vi "例7-1.vi"() -> ()   [LabVIEW 2017]
panel:
  out "7（X0=10，dx=2，Y）多条曲线":cluster{i32, i32, cluster{dbl[]}[]}(graph)
  out "6（X0=10，dx=2，Y）多条曲线":cluster{i32, i32, dbl[][]}(graph)
  out "5（X0=10，dx=2，Y）多条曲线":cluster{i32, i32, dbl[]}[](graph)
  out "4（X0=10，dx=2，Y）单条曲线":cluster{i32, i32, dbl[]}(graph)
  out "3(Y)多条曲线":cluster{dbl[]}[](graph)
  out "2(Y)多条曲线":dbl[][](graph)
  out "1(Y)单条曲线":dbl[](graph)
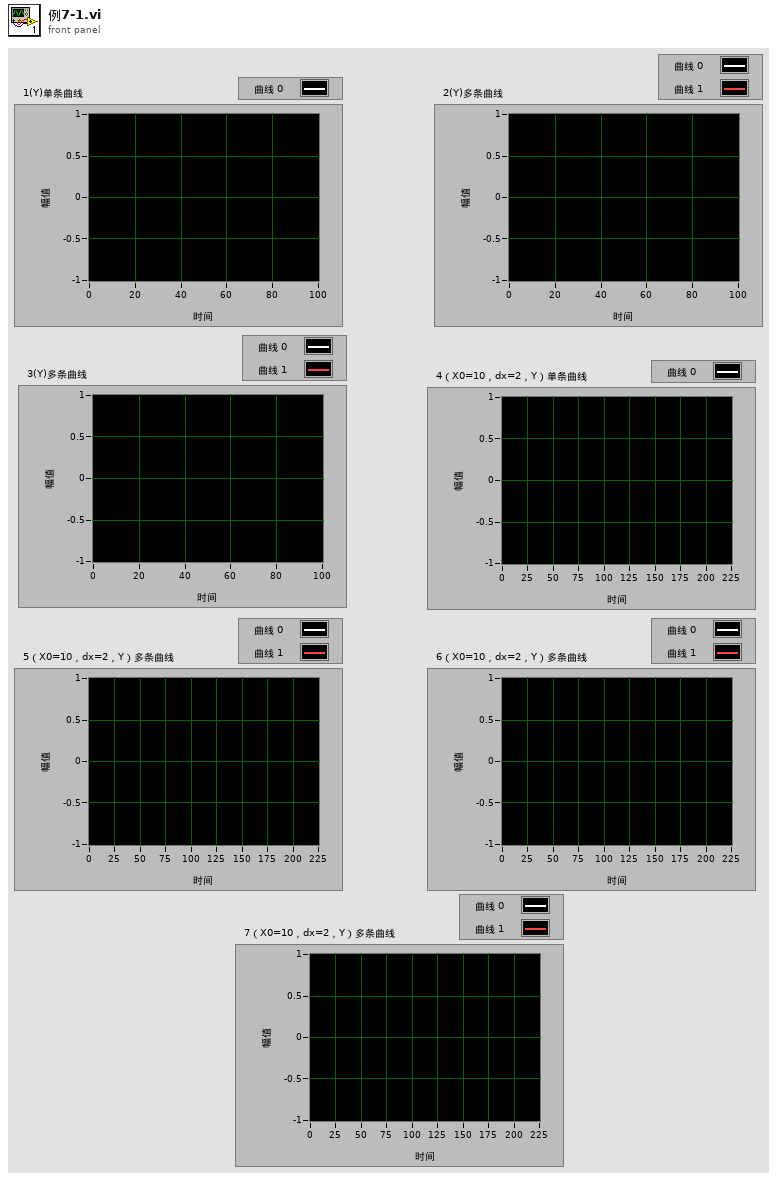
[diagram p1: front panel]
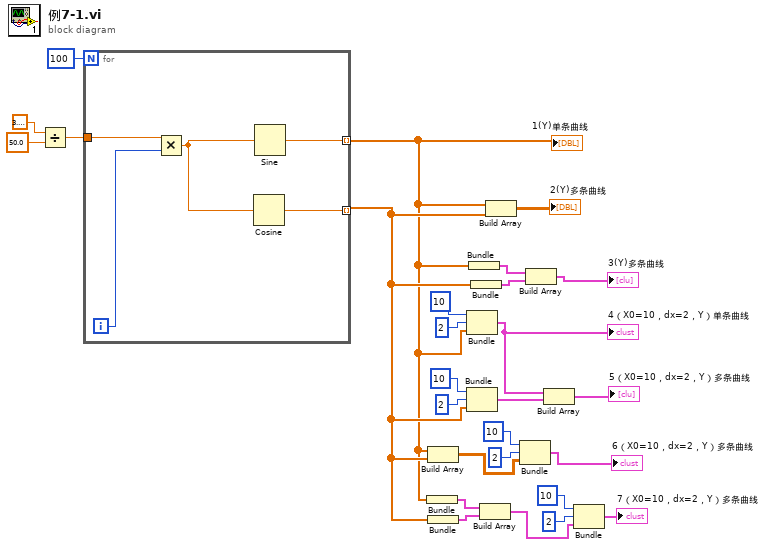
[diagram p0: block diagram]
diagram:
  n1 = Divide(x=3.141592653589793, y=50.0) -> (x/y=w24:dbl)
  n2 = for {
    N: 100 -> [_]
    tunnel: w24 -> [w32]
    tunnel: [w29] -> w1 mode=indexing
    tunnel: [w28] -> w8 mode=indexing
    i -> [w31]
    n3 = Multiply(x=w32, y=w31) -> (x*y=w30:dbl)
    n4 = Cosine(x=w30) -> (cos(x)=w28:dbl)
    n5 = Sine(x=w30) -> (sin(x)=w29:dbl)
  }
  "1(Y)单条曲线" <- w1
  n6 = Bundle(w1) -> (w7:cluster{dbl[]})  [unwired: 1 in]
  n7 = Build Array(w1, w8) -> (w10:dbl[][])
  n8 = Bundle(w8) -> (w6:cluster{dbl[]})  [unwired: 1 in]
  n9 = Bundle(10, 2, w1) -> (w14:cluster{i32, i32, dbl[]})  [unwired: 1 in]
  "4（X0=10，dx=2，Y）单条曲线" <- w14
  n10 = Bundle(10, 2, w8) -> (w15:cluster{i32, i32, dbl[]})  [unwired: 1 in]
  n11 = Bundle(w1) -> (w22:cluster{dbl[]})  [unwired: 1 in]
  n12 = Bundle(w8) -> (w21:cluster{dbl[]})  [unwired: 1 in]
  n13 = Build Array(w7, w6) -> (w3:cluster{dbl[]}[])
  n14 = Build Array(w1, w8) -> (→"2(Y)多条曲线":dbl[][])
  n15 = Bundle(10, 2, w10) -> (→"6（X0=10，dx=2，Y）多条曲线":cluster{i32, i32, dbl[][]})  [unwired: 1 in]
  n16 = Build Array(w22, w21) -> (→"3(Y)多条曲线":cluster{dbl[]}[])
  n17 = Build Array(w14, w15) -> (→"5（X0=10，dx=2，Y）多条曲线":cluster{i32, i32, dbl[]}[])
  n18 = Bundle(10, 2, w3) -> (→"7（X0=10，dx=2，Y）多条曲线":cluster{i32, i32, cluster{dbl[]}[]})  [unwired: 1 in]
